vi "Execute.vi"(8 "error in (no error)":errorcluster, 10 "Abstract Consumer in":refnum<class "Abstract Consumer.lvclass">, 11 "Log Message in":refnum<class "Log Message.lvclass">) -> (0 "error out":errorcluster, 1 "Abstract Response out":refnum<class "Abstract Response Message.lvclass">, 2 "Abstract Consumer out":refnum<class "Abstract Consumer.lvclass">, 3 "Log Message out":refnum<class "Log Message.lvclass">, 4 "Stop?":bool)   [LabVIEW 2020, in "AIM ARINC 664 Engine.lvlib" / "Implementation.lvlib" / "Frame Logging.lvlib" / "Log Message.lvclass"]
uses:
  Log Message.lvclass
  Log Message.lvclass/Log Message.ctl
  Logger Interface/Logger Interface.lvclass
  <vilib>/NI/VeriStand Custom Device Messaging/Consumer/Abstract Consumer/Abstract Consumer.lvclass
  <vilib>/NI/VeriStand Custom Device Messaging/Message/Abstract Response Message/Abstract Response Message.lvclass
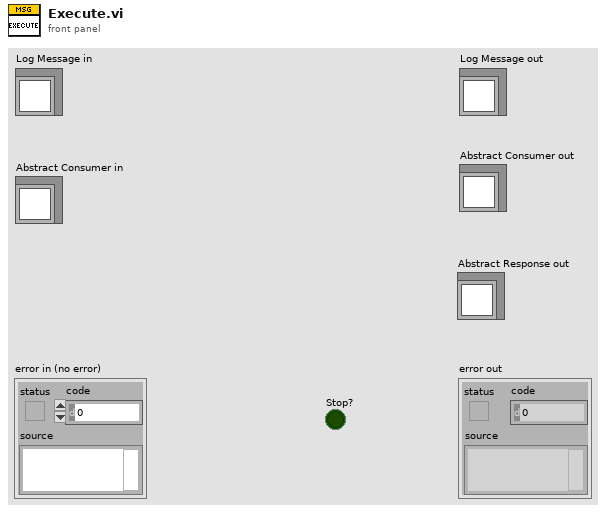
[diagram p1: front panel]
types:
  T1 = typedef "AIM ARINC 664 Engine.lvlib/Implementation.lvlib/Frame Logging.lvlib/Logger Data Reference.ctl" = refnum<data-value>
  T2 = typedef "AIM ARINC 664 Engine.lvlib/Implementation.lvlib/Frame.ctl" = cluster{"FwIrigTime":cluster{"TtHigh":u32, "TtLow":u32}, "Payload":u8[], "Lenght":u32}
  T3 = cluster{"Logger Interface.lvclass":refnum<class "Logger Interface.lvclass">}
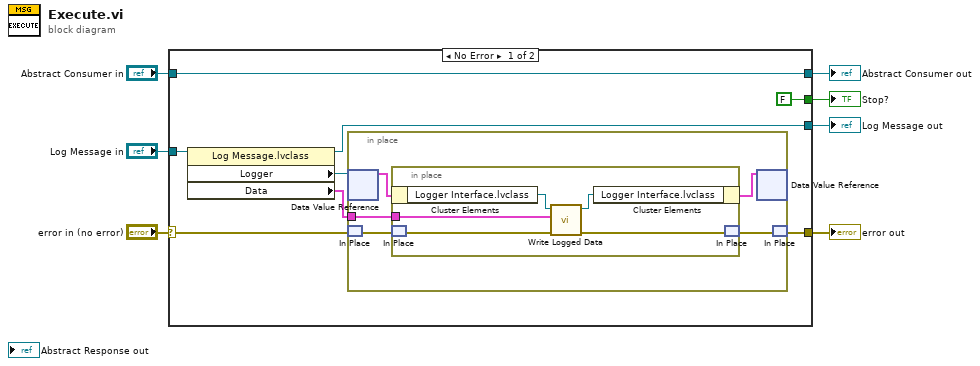
[diagram p0: block diagram]
diagram:
  n1 = case shown="No Error" "error in (no error)" {
    selector: "error in (no error)" -> [w10 w28]
    tunnel: [w9 w28] -> w6
    tunnel: [w8 w27] -> w5
    tunnel: "Log Message in" -> [w13 w27]
    tunnel: [w14 w26] -> w3
    tunnel: "Abstract Consumer in" -> [w14 w26]
    tunnel: [FALSE ("Stop?") _] -> w1
    frame No Error {
      n2 = property class="Log Message.lvclass"(reference=w13) -> (reference out=w8:refnum<class "Log Message.lvclass">, "Logger"=w12:T1, "Data"=w11:T2[])  [unwired: 1 in, 1 out]
      n3 = in-place {
        in-place-border: w11 -> [w19]
        n4 = in-place-dvr #1(w12) -> (w20:T3)  [unwired: 1 out]
        n5 = in-place-match #2(w10) -> (w18:errorcluster)
        n6 = in-place {
          in-place-border: w19 -> [w24]
          n7 = in-place-cluster #3(w20) -> ("Logger Interface.lvclass"=w25:refnum<class "Logger Interface.lvclass">)
          n8 = in-place-match #4(w18) -> (w23:errorcluster)
          n9 = call-dynamic "Write Logged Data.vi"("error in (no error)"=w23, "Data"=w24, "Logger Interface in"=w25) -> ("error out"=w22:errorcluster, "Logger Interface out"=w21:refnum<class "Logger Interface.lvclass">)  [unwired: 7 in]
          n10 = in-place-cluster #3("Logger Interface.lvclass"=w21) -> (w17:T3)
          n11 = in-place-match #4(w22) -> (w16:errorcluster)
        }
        n12 = in-place-dvr #1(w17) -> ()  [unwired: 2 out]
        n13 = in-place-match #2(w16) -> (w9:errorcluster)
      }
    }
    frame Error {
    }
  }
  "error out" <- w6
  "Log Message out" <- w5
  "Abstract Consumer out" <- w3
  "Stop?" <- w1
